vi "模块配置写入.vi"(8 "error in (no error)":errorcluster caption="错误输入（无错误）") -> (0 "错误输出":errorcluster)   [LabVIEW 2016, in "斯坦道总磷.lvlib"]
uses:
  <vilib>/Utility/config.llb/NI_LVConfig.lvlib
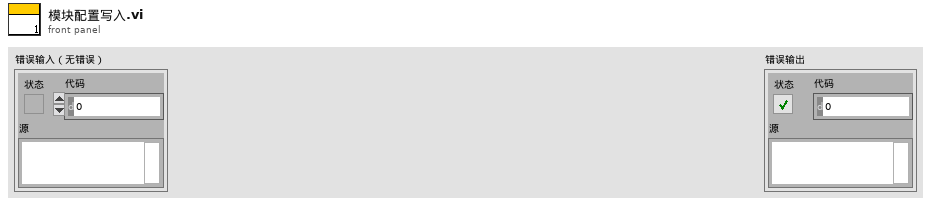
[diagram p1: front panel]
types:
  T1 = typedef "NI_LVConfig.lvlib/Config Data RefNum.ctl" = refnum<k1>
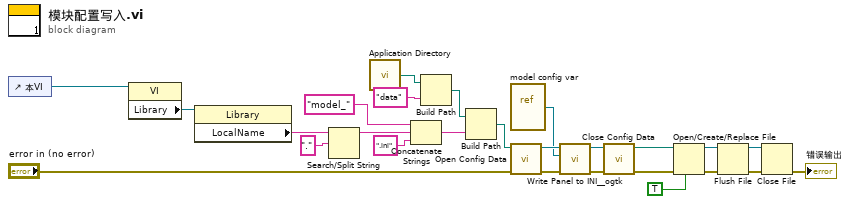
[diagram p0: block diagram]
diagram:
  n1 = control-ref of="本VI"() -> (w8:refnum<vi>)
  n2 = property class="VI"(reference=w8) -> ("Library"=w9:refnum<vi>)  [unwired: 1 in, 2 out]
  n3 = property class="Library"(reference=w9) -> ("LocalName"=w7:string)  [unwired: 1 in, 2 out]
  n4 = Search/Split String(string=w7, search string/char (-)="." ("搜索字符串/字符(-)")) -> (substring before match=w5:string)  [unwired: 1 in, 2 out]
  n5 = call <vilib>:"Application Directory.vi"() -> ("Application Directory"=w11:path)
  n6 = Concatenate Strings("model_" ("字符串"), w5, ".ini" ("字符串")) -> (w4:string)
  n7 = Build Path(base path=w11, name or relative path="data" ("名称或相对路径")) -> (appended path=w10:path)
  n8 = Build Path(base path=w10, name or relative path=w4) -> (appended path=w1:path)
  n9 = vi-ref "model config var.vi"() -> (w25:refnum<vi>)
  n10 = call <vilib>:"Open Config Data.vi"("error in (no error)"="error in (no error)", "configuration file path"=w1) -> ("error out"=w23:errorcluster, "refnum"=w26:T1)  [unwired: 7 in, 1 out]
  n11 = call <userlib>:"Write Panel to INI__ogtk.vi"("error in (no error)"=w23, "VI ref"=w25, "refnum"=w26) -> ("error out"=w22:errorcluster, "refnum out"=w24:T1)  [unwired: 7 in]
  n12 = call <vilib>:"Close Config Data.vi"("error in (no error)"=w22, "refnum"=w24) -> ("error out"=w17:errorcluster, "file path"=w16:path)  [unwired: 8 in]
  n13 = Open/Create/Replace File(file path (use dialog)=w16, error in=w17, disable buffering (F)=TRUE ("禁用缓存(F)")) -> (refnum out=w20:refnum<file>, error out=w21:errorcluster)  [unwired: 3 in, 1 out]
  n14 = Flush File(refnum=w20, error in=w21) -> (refnum out=w19:refnum<file>, error out=w18:errorcluster)
  n15 = Close File(refnum=w19, error in=w18) -> (error out=→"错误输出":errorcluster)  [unwired: 1 out]
